vi "Generate Library Icon.vi"(8 "error in (no error)":errorcluster, 9 "Overlay Text":string, 10 "Library":refnum<vi>, 11 "Process Generator In":refnum<class "Process Generator.lvclass">) -> (0 "error out":errorcluster, 2 "Library Out":refnum<vi>, 3 "Process Generator Out":refnum<class "Process Generator.lvclass">)   [LabVIEW 2020, in "Process Generation.lvlib" / "Process Generator.lvclass"]
uses:
  Process Generator.lvclass
  <vilib>/LabVIEW Icon API/lv_icon/Classes/Icon/Icon.lvclass
  <vilib>/LabVIEW Icon API/API_Rectangle Dimension.ctl
  <vilib>/LabVIEW Icon API/API_Text.ctl
  Process Generator.lvclass/Process Generator.ctl
  <vilib>/LabVIEW Icon API/LabVIEW Icon API.lvlib
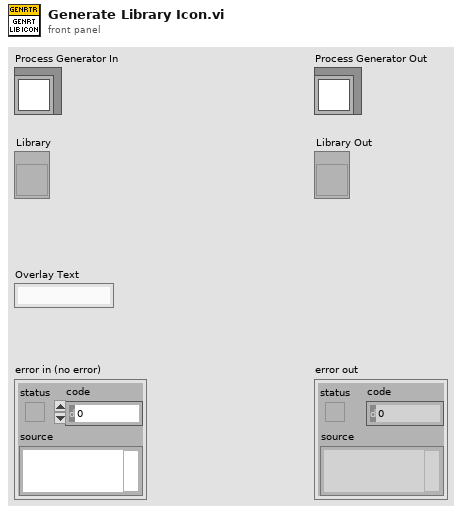
[diagram p1: front panel]
types:
  T1 = typedef "LabVIEW Icon API.lvlib/API_Text.ctl" = cluster{"Line 1 text":string, "Line 2 text":string, "Line 3 text":string, "Line 4 text":string}
  T2 = typedef "LabVIEW Icon API.lvlib/API_Rectangle Dimension.ctl" = cluster{"Width":i16, "Height":i16}
  T3 = typedef "LabVIEW Icon API.lvlib/API_Rectangle Colors.ctl" = cluster{"Border":u32, "Background":u32}
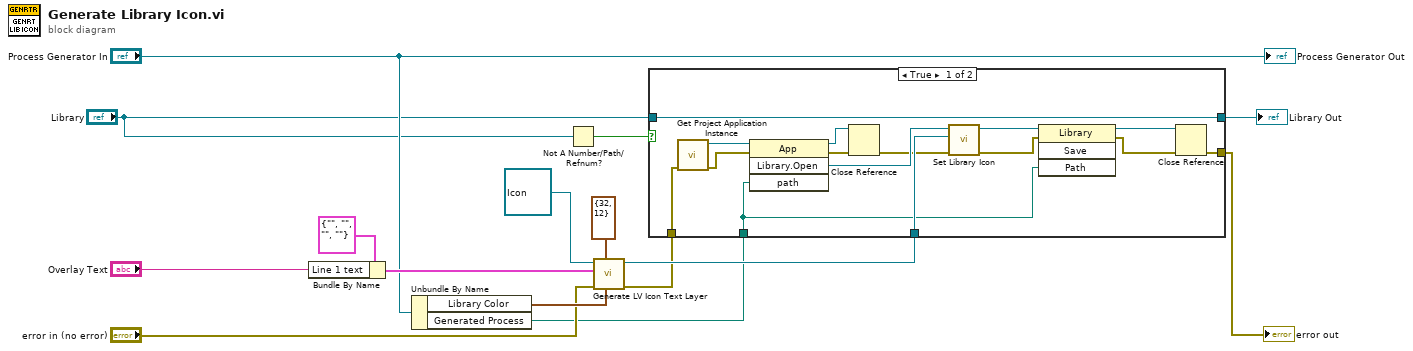
[diagram p0: block diagram]
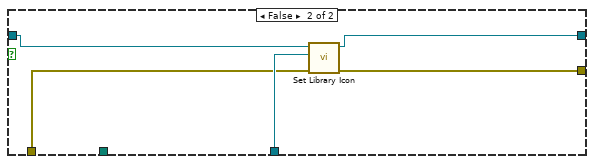
[diagram p2: hidden frame]
diagram:
  n1 = Bundle By Name(cluster=T1 {"Line 1 text"="", "Line 2 text"="", "Line 3 text"="", "Line 4 text"=""} ("Text"), "Line 1 text"="Overlay Text") -> (w11:T1)
  n2 = Unbundle By Name("Process Generator In") -> ("Library Color"=w8:T3, "Generated Process"=w6:path)
  n3 = Not A Number/Path/Refnum?(number/path/refnum="Library") -> (NaN/Path/Refnum?=w3:bool)
  n4 = call <vilib>:"Generate LV Icon Text Layer.vi"("Rectangle colors (black, white)"=w8, "Rectangle dimension (32,32)"=T2 {"Width"=32, "Height"=12}, "error in (no error)"="error in (no error)", "Text"=w11, "Icon in"=refnum<class "Icon.lvclass"> refnum ("Icon.lvclass in")) -> ("error out"=w4:errorcluster, "Icon out"=w12:refnum<class "Icon.lvclass">)  [unwired: 5 in]
  n5 = case shown="True" w3 {
    tunnel: w12 -> [w30 w34]
    tunnel: w6 -> [w16 _]
    tunnel: [w26 w35] -> w5
    tunnel: w4 -> [w24 w33]
    tunnel: "Library" -> [w20 w32]
    tunnel: [w20 w31] -> w1
    frame True {
      n6 = call "Get Project Application Instance.vi"("error in (no error)"=w24) -> ("error out"=w28:errorcluster, "Application out"=w29:refnum<vi>)  [unwired: 9 in]
      n7 = invoke class="App" method="Library.Open"(reference=w29, error in=w28, "path"=w16) -> (reference out=w21:refnum<vi>, error out=w23:errorcluster, "Open Library"=w27:refnum<vi>)  [unwired: 1 in, 1 out]
      n8 = Close Reference(reference=w21, error in (no error)=w23) -> (error out=w22:errorcluster)
      n9 = call <vilib>:"Set Library Icon.vi"("error in (no error)"=w22, "Icon"=w30, "Library Refnum in"=w27) -> ("error out"=w18:errorcluster, "Library Refnum out"=w25:refnum<vi>)  [unwired: 7 in]
      n10 = invoke class="Library" method="Save"(reference=w25, error in=w18, "Path"=w16) -> (reference out=w19:refnum<vi>, error out=w17:errorcluster)  [unwired: 1 in, 2 out]
      n11 = Close Reference(reference=w19, error in (no error)=w17) -> (error out=w26:errorcluster)
    }
    frame False {
      n12 = call <vilib>:"Set Library Icon.vi"("error in (no error)"=w33, "Icon"=w34, "Library Refnum in"=w32) -> ("error out"=w35:errorcluster, "Library Refnum out"=w31:refnum<vi>)  [unwired: 7 in]
    }
  }
  "error out" <- w5
  "Library Out" <- w1
  "Process Generator Out" <- "Process Generator In"
